vi "Get Excel All SheetNames.vi"(8 "error in (no error)":errorcluster, 11 "path":path) -> (0 "error out":errorcluster, 2 "SheetNames(\"\")":string[](array[string]))   [LabVIEW 2015]
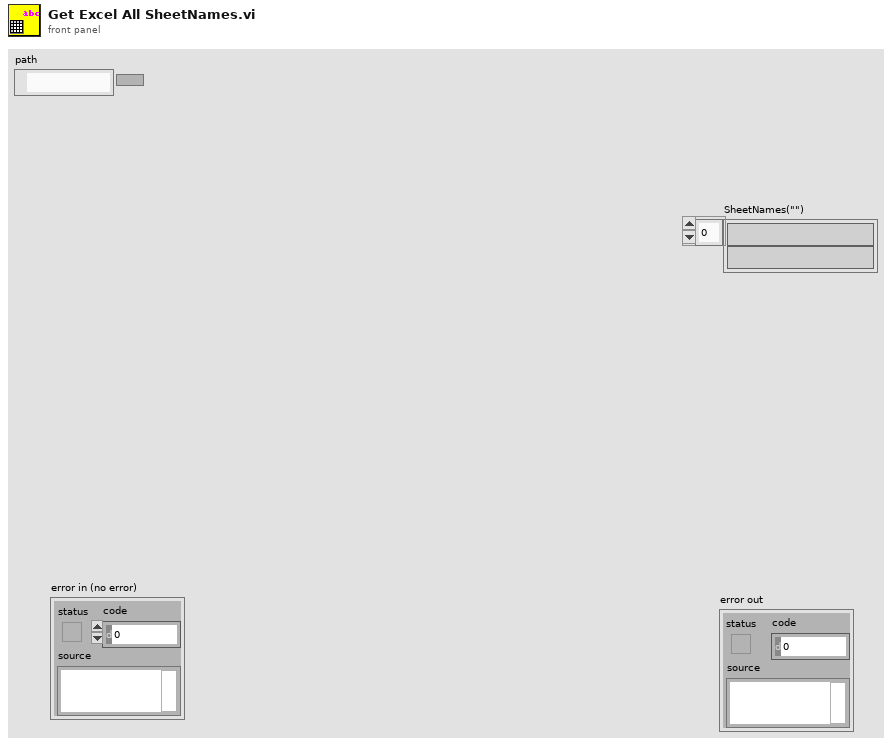
[diagram p1: front panel]
types:
  T1 = cluster{"Excel._Application":refnum<k7>, "Workbooks":refnum<k7>}
  T2 = cluster{"Excel._Application":refnum<k7>, "Workbooks":refnum<k7>, "Open":refnum<k7>}
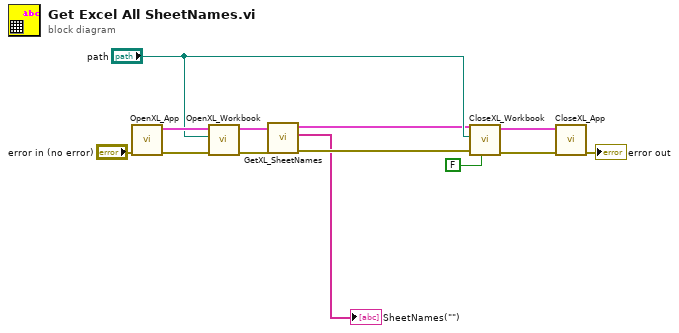
[diagram p0: block diagram]
diagram:
  n1 = call "OpenXL_App.vi"("error in (no error)"="error in (no error)") -> ("error out"=w12:errorcluster, "Refnum Cluster"=w13:T1)  [unwired: 9 in]
  n2 = call "OpenXL_Workbook.vi"("error in"=w12, "path"="path", "Refnum Cluster In"=w13) -> ("error out"=w7:errorcluster, "Refnum Cluster Out"=w8:T2)  [unwired: 7 in]
  n3 = call "GetXL_SheetNames.vi"("error in (no error)"=w7, "Refnum Cluster In"=w8) -> ("error out"=w4:errorcluster, "SheetNames(\"\")"=→"SheetNames(\"\")":string[], "Refnum Cluster Out"=w5:T2)  [unwired: 7 in]
  n4 = call "CloseXL_Workbook.vi"("Save? (F)"=FALSE, "error in (no error)"=w4, "path"="path", "Refnum Cluster In"=w5) -> ("error out"=w11:errorcluster, "Refnum Cluster Out"=w10:T1)  [unwired: 6 in]
  n5 = call "CloseXL_App.vi"("error in (no error)"=w11, "Refnum Cluster In"=w10) -> ("error out"=→"error out":errorcluster)  [unwired: 9 in]
